vi "Variant to string.vi"(8 "error in (no error)":errorcluster, 11 "Variant":variant) -> (0 "error out":errorcluster, 3 "String":string)   [LabVIEW 2020, in "LUnit Test Case.lvclass"]
uses:
  LUnit Test Case.lvclass
  LUnit Test Case.lvclass/LUnit Test Case.ctl
  <vilib>/Utility/Data Type/NI_Data Type.lvlib
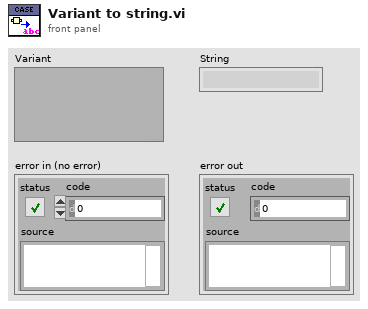
[diagram p1: front panel]
types:
  T1 = typedef "NI_Data Type.lvlib/Data Type.ctl" = enum8{"Invalid Type", "Void", "I8", "I16", "I32", "I64", "U8", "U16", "U32", "U64", "Single Float", "Double Float", "Extended Float", "Single Complex", "Double Complex", "Extended Complex", "Enum U8", "Enum U16", "Enum U32", "Enum U64", "Single Float With Unit", "Double Float With Unit", "Extended Float With Unit", "Single Complex with Unit", "Double Complex with Unit", "Extended Complex with Unit", "Boolean", "String", "Path", "Picture", "Tag", "Array", "Cluster", "Variant", "LV Variant", "Waveform", "Timestamp", "Digital Waveform", "Digital Data", "ExpressData", "Refnum", "External Data", "VI", "Poly VI", "LabVIEW Class Instance", "Fixed Point", "Set Collection", "Map Collection"}
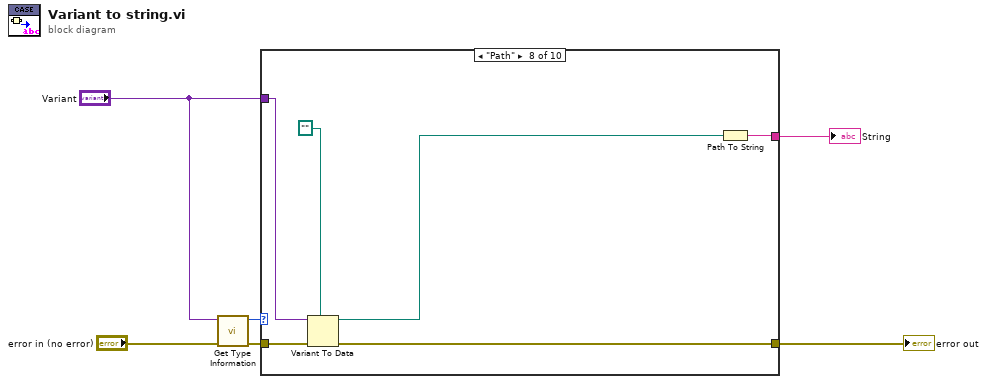
[diagram p0: block diagram]
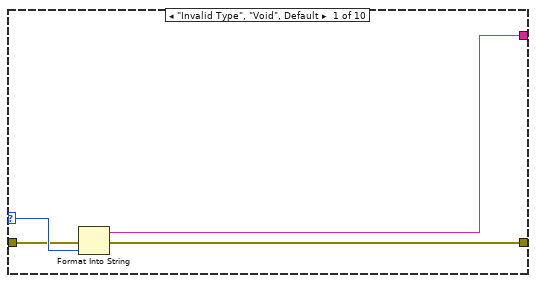
[diagram p2: hidden frame]
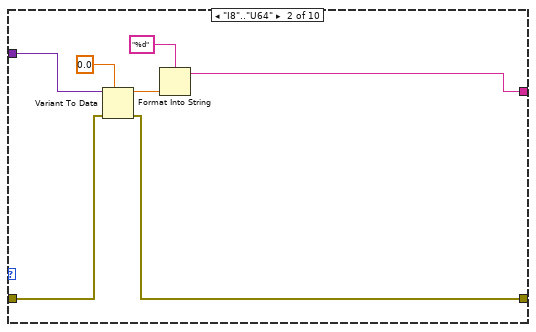
[diagram p3: hidden frame]
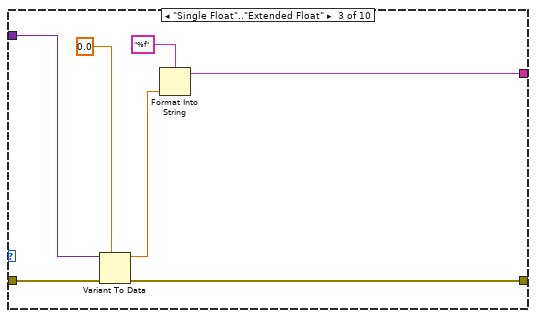
[diagram p4: hidden frame]
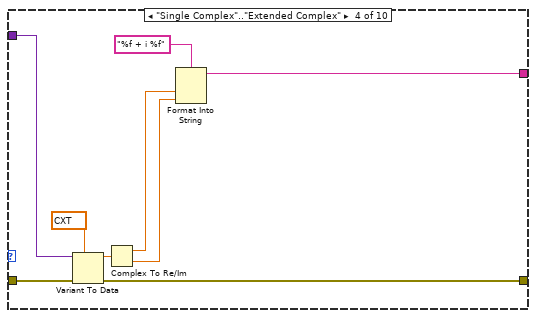
[diagram p5: hidden frame]
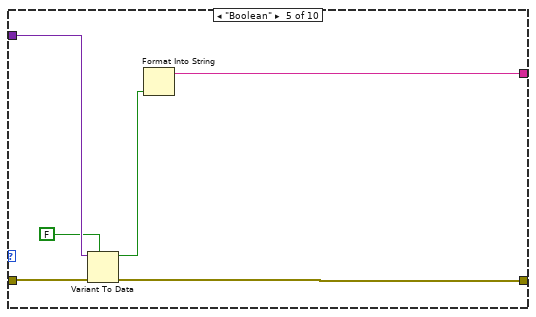
[diagram p6: hidden frame]
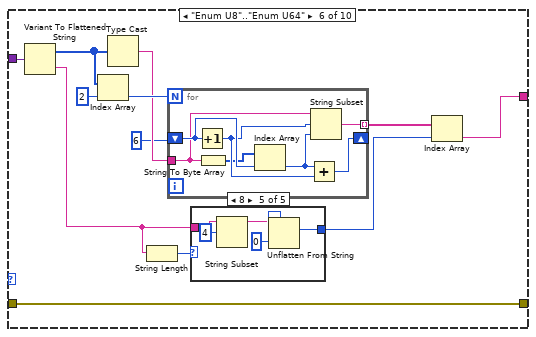
[diagram p7: hidden frame]
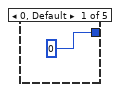
[diagram p8: hidden frame]
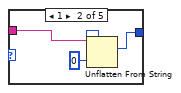
[diagram p9: hidden frame]
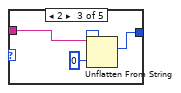
[diagram p10: hidden frame]
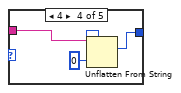
[diagram p11: hidden frame]
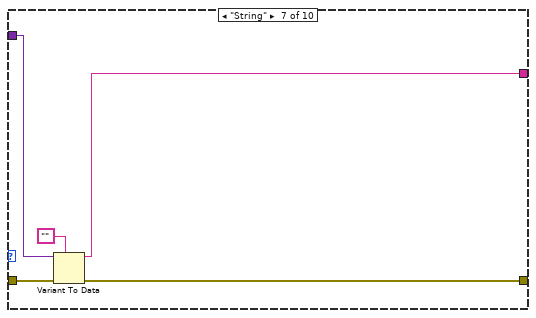
[diagram p12: hidden frame]
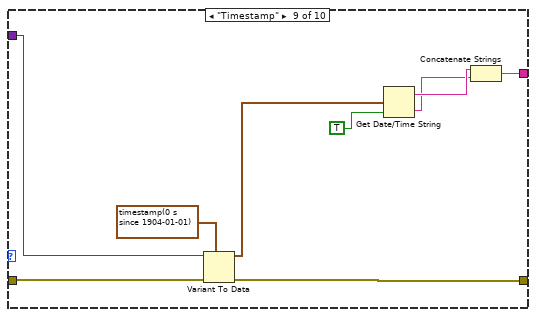
[diagram p13: hidden frame]
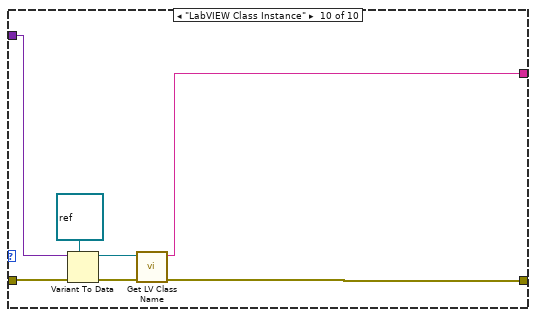
[diagram p14: hidden frame]
diagram:
  n1 = call <vilib>:"Get Type Information.vi"("error in (no error)"="error in (no error)", "variant"="Variant") -> ("error out"=w4:errorcluster, "type"=w5:T1)  [unwired: 5 in, 3 out]
  n2 = case shown="\"Path\"" w5 {
    selector: w5 -> [w10 _ _ _ _ _ _ _ _ _]
    tunnel: "Variant" -> [_ w17 w24 w33 w38 w50 w77 w83 w92 w100]
    tunnel: [w7 w13 w20 w31 w35 w40 w75 w81 w87 w94] -> w6
    tunnel: w4 -> [w9 w12 w19 w30 w39 w51 w78 w84 w93 w98]
    tunnel: [w8 w11 w18 w25 w34 w51 w74 w79 w86 w95] -> w3
    frame "Invalid Type", "Void", Default {
      n3 = Format Into String(error in=w9, w10) -> (resulting string=w7:string, error out=w8:errorcluster)  [unwired: 2 in]
    }
    frame "I8".."U64" {
      n4 = Variant To Data(error in=w12, type=0.0 ("double precision float"), Variant=w17) -> (data=w15:dbl, error out=w11:errorcluster)
      n5 = Format Into String(format string="%d", w15) -> (resulting string=w13:string)  [unwired: 2 in, 1 out]
    }
    frame "Single Float".."Extended Float" {
      n6 = Variant To Data(error in=w19, type=0.0 ("double precision float"), Variant=w24) -> (data=w22:dbl, error out=w18:errorcluster)
      n7 = Format Into String(format string="%f", w22) -> (resulting string=w20:string)  [unwired: 2 in, 1 out]
    }
    frame "Single Complex".."Extended Complex" {
      n8 = Variant To Data(error in=w30, type=cxt 0.0+0.0i, Variant=w33) -> (data=w28:cxt, error out=w25:errorcluster)
      n9 = Complex To Re/Im(x + iy=w28) -> (x=w27:ext, y=w26:ext)
      n10 = Format Into String(format string="%f + i %f", w27, w26) -> (resulting string=w31:string)  [unwired: 2 in, 1 out]
    }
    frame "Boolean" {
      n11 = Variant To Data(error in=w39, type=FALSE, Variant=w38) -> (data=w36:bool, error out=w34:errorcluster)
      n12 = Format Into String(w36) -> (resulting string=w35:string)  [unwired: 3 in, 1 out]
    }
    frame "Enum U8".."Enum U64" {
      n13 = Variant To Flattened String(Variant=w50) -> (data string=w43:string, 1:w49:i16[])
      n14 = Index Array(array=w49, index=2) -> (element=w47:i16)
      n15 = Type Cast(x=w49) -> (*(type *) &x=w46:string)  [unwired: 1 in]
      n16 = String Length(string=w43) -> (length=w44:i32)
      n17 = for {
        N: w47 -> [_]
        tunnel: w46 -> [w70]
        shift-right: [w71] -> _
        shift-left: 6 -> [w72]
        tunnel: [w73] -> w42 mode=indexing
        n18 = Increment(x=w72) -> (x+1=w68:i32)
        n19 = String To Byte Array(string=w70) -> (unsigned byte array=w67:u8[])
        n20 = Index Array(array=w67, index=w72) -> (element=w69:u8)
        n21 = Add(x=w69, y=w68) -> (x+y=w71:i32)
        n22 = String Subset(string=w70, offset (0)=w68, length (rest)=w69) -> (substring=w73:string)
      }
      n23 = case shown="8" w44 {
        tunnel: w43 -> [_ w55 w58 w61 w62]
        tunnel: [u32 0 ("U32") w53 w56 w59 w65] -> w41
        frame 0, Default {
        }
        frame 1 {
          n24 = Unflatten From String(type=u8 0 ("U8"), binary string=w55) -> (value=w53:u8)  [unwired: 3 in, 2 out]
        }
        frame 2 {
          n25 = Unflatten From String(type=u16 0 ("U16"), binary string=w58) -> (value=w56:u16)  [unwired: 3 in, 2 out]
        }
        frame 4 {
          n26 = Unflatten From String(type=u32 0 ("U32"), binary string=w61) -> (value=w59:u32)  [unwired: 3 in, 2 out]
        }
        frame 8 {
          # "Enum 64"
          n27 = String Subset(string=w62, offset (0)=4) -> (substring=w63:string)  [unwired: 1 in]
          n28 = Unflatten From String(type=u32 0 ("U32"), binary string=w63) -> (value=w65:u32)  [unwired: 3 in, 2 out]
        }
      }
      n29 = Index Array(array=w42, index=w41) -> (element=w40:string)
    }
    frame "String" {
      n30 = Variant To Data(error in=w78, type="", Variant=w77) -> (data=w75:string, error out=w74:errorcluster)
    }
    frame "Path" {
      n31 = Variant To Data(error in=w84, type=path "", Variant=w83) -> (data=w80:path, error out=w79:errorcluster)
      n32 = Path To String(path=w80) -> (string=w81:string)
    }
    frame "Timestamp" {
      n33 = Variant To Data(error in=w93, type=timestamp(0 s since 1904-01-01), Variant=w92) -> (data=w90:timestamp, error out=w86:errorcluster)
      n34 = Get Date/Time String(seconds (now)=w90, want seconds? (F)=TRUE) -> (date string=w89:string, time string=w88:string)  [unwired: 1 in]
      n35 = Concatenate Strings(w89, w88) -> (w87:string)
    }
    frame "LabVIEW Class Instance" {
      n36 = Variant To Data(error in=w98, type=refnum<class> refnum ("object"), Variant=w100) -> (data=w97:refnum<class>, error out=w96:errorcluster)
      n37 = call <vilib>:"Get LV Class Name.vi"("error in (no error)"=w96, "object"=w97) -> ("error out"=w95:errorcluster, "class name"=w94:string)  [unwired: 8 in]
    }
  }
  "error out" <- w3
  "String" <- w6
